vi "SQLite Edit Subcategory Test.vi"(7 "Test DB Set Up Command":string, 8 "Error In (no error)":errorcluster, 11 "SQLite DB Operator In":refnum<class "SQLite DB Operator.lvclass">) -> (0 "Error Out":errorcluster, 3 "SQLite DB Operator Out":refnum<class "SQLite DB Operator.lvclass">)   [LabVIEW 2023]
uses:
  Clasess/SQLite DB Operator/SQLite DB Operator.lvclass
  Clasess/DB Records/Expenses Tracker Subcategory/Public/Ctrls/Subcategory.ctl
  Clasess/DB Records/Expenses Tracker Subcategory/Expenses Tracker Subcategory.lvclass
  H:/Desktop/LabVIEW/LabView Repo/Expenses-Tracker-DB-Operator/Interfaces/Expenses Tracker Record/Expenses Tracker Record.lvclass
  Support/Editing/Edit Record Assert Error.vi
  Support/Editing/Edit Record Assert Not Error.vi
  <vilib>/drjdpowell/SQLite Library/SQL Connection/Execute SQL (1D Cluster).vi
  <vilib>/addons/_JKI Toolkits/Caraya/classes/Test/Test.lvclass
  <vilib>/drjdpowell/SQLite Library/SQLite.lvlib
  H:/Desktop/LabVIEW/LabView Repo/Expenses-Tracker-DB-Operator/Clasess/DB Records/Expenses Tracker Subcategory/Expenses Tracker Subcategory.lvclass
  <vilib>/drjdpowell/SQLite Library/SQL Connection/Connection.lvclass
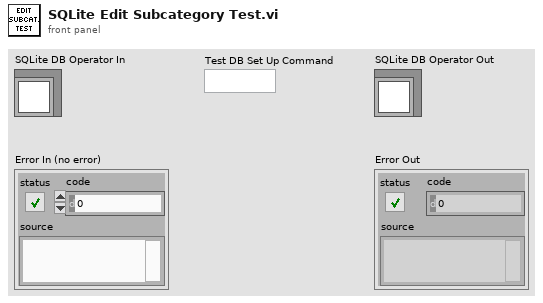
[diagram p1: front panel]
types:
  T1 = typedef "Expenses Tracker Subcategory.lvclass/Subcategory.ctl" = cluster{"ID":u32, "Name":string, "Category":u32}
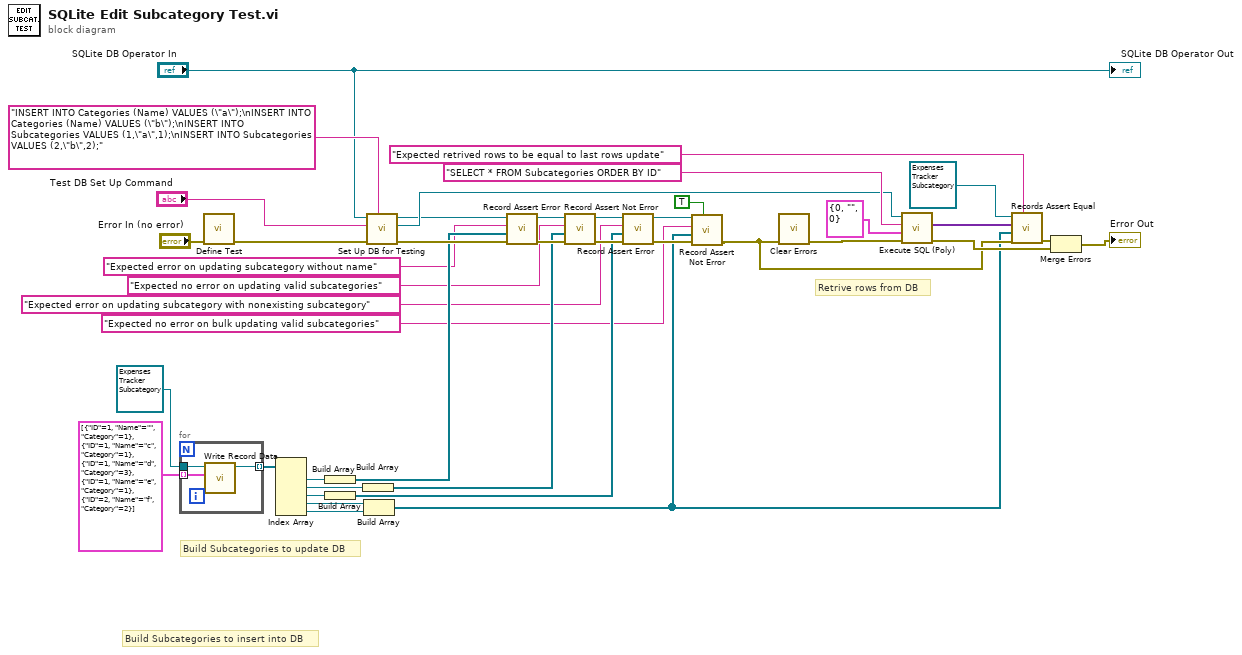
[diagram p0: block diagram]
diagram:
  # "Retrive rows from DB"
  # "Build Subcategories to update DB"
  # "Build Subcategories to insert into DB"
  n1 = for {
    tunnel: T1[] [{"ID"=1, "Name"="", "Category"=1}, {"ID"=1, "Name"="c", "Category"=1}, {"ID"=1, "Name"="d", "Category"=3}, {"ID"=1, "Name"="e", "Category"=1}, {"ID"=2, "Name"="f", "Category"=2}] ("Array") -> [w44] mode=indexing
    tunnel: refnum<class "Expenses Tracker Subcategory.lvclass"> refnum ("Expenses Tracker Category") -> [w43]
    tunnel: [w42] -> w38 mode=indexing
    n2 = call-dynamic "Write Record Data.vi"("Record"=w44, "Expenses Tracker Subcategory In"=w43) -> ("Expenses Tracker Subcategory Out"=w42:refnum<class "Expenses Tracker Subcategory.lvclass">)  [unwired: 8 in, 1 out]
  }
  n3 = call <vilib>:"Define Test.vi"("error in (no error)"="Error In (no error)") -> ("error out"=w31:errorcluster)  [unwired: 9 in, 1 out]
  n4 = Index Array(array=w38) -> (element #1=w37:refnum<class "Expenses Tracker Subcategory.lvclass">, element #2=w36:refnum<class "Expenses Tracker Subcategory.lvclass">, element #3=w6:refnum<class "Expenses Tracker Subcategory.lvclass">, element #4=w4:refnum<class "Expenses Tracker Subcategory.lvclass">, element #5=w3:refnum<class "Expenses Tracker Subcategory.lvclass">)  [unwired: 5 in]
  n5 = Build Array(w37) -> (w19:refnum<class "Expenses Tracker Subcategory.lvclass">[])
  n6 = Build Array(w6) -> (w5:refnum<class "Expenses Tracker Subcategory.lvclass">[])
  n7 = Build Array(w36) -> (w12:refnum<class "Expenses Tracker Subcategory.lvclass">[])
  n8 = Build Array(w4, w3) -> (w1:refnum<class "Expenses Tracker Subcategory.lvclass">[])
  n9 = call "Set Up DB for Testing.vi"("Additional Set Up Commands"="INSERT INTO Categories (Name) VALUES (\"a\");\nINSERT INTO Categories (Name) VALUES (\"b\");\nINSERT INTO Subcategories VALUES (1,\"a\",1);\nINSERT INTO Subcategories VALUES (2,\"b\",2);", "Error In (no error)"=w31, "Test DB Set Up Command"="Test DB Set Up Command", "SQLite DB Operator In"="SQLite DB Operator In") -> ("Error Out"=w20:errorcluster, "SQLite Connection"=w33:refnum<class "Connection.lvclass">, "SQLite DB Operator Out"=w18:refnum<class "SQLite DB Operator.lvclass">)  [unwired: 5 in]
  n10 = call-poly "Record Assert Error.vi"("Error In"=w20, "Records"=w19, "Assertion Label"="Expected error on updating subcategory without name" ("Label (VI Title)"), "SQLite DB Operator In"=w18) -> ("Error Out"=w23:errorcluster, "SQLite DB Operator Out"=w24:refnum<class "SQLite DB Operator.lvclass">)  [unwired: 6 in]
  n11 = call-poly "Record Assert Not Error.vi"("Error In"=w23, "Records"=w12, "Assertion Label"="Expected no error on updating valid subcategories" ("Label (VI Title)"), "SQLite DB Operator In"=w24) -> ("Error Out"=w21:errorcluster, "SQLite DB Operator Out"=w22:refnum<class "SQLite DB Operator.lvclass">)  [unwired: 6 in]
  n12 = call-poly "Record Assert Error.vi"("Error In"=w21, "Records"=w5, "Assertion Label"="Expected error on updating subcategory with nonexisting subcategory" ("Label (VI Title)"), "SQLite DB Operator In"=w22) -> ("Error Out"=w10:errorcluster, "SQLite DB Operator Out"=w9:refnum<class "SQLite DB Operator.lvclass">)  [unwired: 6 in]
  n13 = call-poly "Record Assert Not Error.vi"("Bulk Update?"=TRUE ("Bulk Insert?"), "Error In"=w10, "Records"=w1, "Assertion Label"="Expected no error on bulk updating valid subcategories" ("Label (VI Title)"), "SQLite DB Operator In"=w9) -> ("Error Out"=w7:errorcluster)  [unwired: 5 in, 1 out]
  n14 = call <vilib>:"Clear Errors.vi"("error in (no error)"=w7) -> ("error out"=w28:errorcluster)  [unwired: 5 in, 1 out]
  n15 = call-poly <vilib>:"Execute SQL (Poly).vi"("error in (no error)"=w28, "Cluster (or Array of Clusters)"=T1 {"ID"=0, "Name"="", "Category"=0} ("Subcategory"), "SQL"="SELECT * FROM Subcategories ORDER BY ID", "SQLite Connection in"=w33) -> ("error out"=w15:errorcluster, "Result Set (Array of Clusters)"=w27:variant[])  [unwired: 5 in, 1 out]
  n16 = call "Records Assert Equal.vi"("Assertion Label"="Expected retrived rows to be equal to last rows update" ("Label (VI Title)"), "Error In"=w7, "Correct Records"=w1, "Typedef Records"=w27, "Expenses Tracker Record In"=refnum<class "Expenses Tracker Subcategory.lvclass"> refnum ("Expenses Tracker Category")) -> ("Error Out"=w16:errorcluster)  [unwired: 6 in]
  n17 = Merge Errors(w16, w15) -> (→"Error Out":errorcluster)
  "SQLite DB Operator Out" <- "SQLite DB Operator In"
